vi "STAGE+mono+counter_edit24.vi"() -> ()   [LabVIEW 2017]
panel:
  out "Timeout":bool
  out "PROGRESS":sgl(slide) max=10 step=10 scale=0.0..1.0
  in  "?":enum32{"Scan Data", "Scans", "RT Data"}(tab)
  out "Spectrum":cluster{dbl[], dbl[]}(graph)
  out "Decay":cluster{dbl[], dbl[]}[](graph)
  in  "Collect Data!":bool
  out "Waveform Graph":waveform(dbl)[](graph)
  out "?":sgl(knob) scale=0.0..1000000.0
  out "Photon Counts":sgl
  in  "Wavelength":sgl
  in  "Show Real Time Data":bool
  in  "?":enum32{"DELAY", "COUNTER", "MONO", "PLOT"}(tab)
  in  "Data File Path":path
  out "Final time [ps]":sgl
  out "Current time [ps]":sgl
  out "Initial time [ps]":sgl
  in  "Set this as t0":bool
  in  "Axis":i64=1
  in  "Motor ON":bool
  in  "Motor OFF":bool
  out "Current Position [mm]":sgl
  out "Final Position [mm]":sgl
  in  "Data Points":sgl=100.0
  out "Current Point":sgl
  in  "Step Size [um]":sgl=10.0
  in  "Target [mm]":sgl format="%.3f"
  in  "Move":bool
  out "Initial position [mm]":sgl
  in  "GPIB address":string="23"
  in  "Count Mode":sgl(ring) items=["A,B for Preset T", "A-B for Preset T", "A+B for Preset T", "A for Preset B"]
  in  "Trigger mode":u16(ring) items=["10 MHz"=0, "Input 2"=2, "Input T"=3]
  in  "Channel A Input":sgl(ring)=1.0 items=["10 MHz", "Input 1"]
  in  "Channel B Input":u16(ring)=2 items=["Input 1"=1, "Input 2"=2]
  in  "Number of Measurements\n to take at one point/ Number of Periods":sgl=1.0 min=1 max=2000 step=1
  in  "Time between measurements\n at one point (s)/Dwell Time":sgl=0.002 min=0.002 max=60 step=0.001
  in  "gate mode (CW:0)":sgl(slide) scale=0.0..2.0 scale format="%.2f"
  out "Counts":sgl
  in  "Integrating time \nin 10^-7 sec":sgl=10000000.0
  in  "Discriminator Level (mV)":dbl min=-300.0 max=300.0 step=0.2
  in  "Discriminator Slope":bool
  in  "Channel":i16 min=0 max=2 step=1
  out "Current Units \n0=microns\n1=nanometers\n2=angstroms":dbl
  out "Grating #":sgl
  out "Blaze angle":sgl
  out "Grooves/mm":sgl
  out "Mono port":T1(ring)
  out "Time delay":sgl=450000.0 min=1
  in  "Step size":sgl=10.0 min=0
  in  "Scan to":sgl=4000.0
  in  "Scan from":sgl=2600.0
  out "Current wavelength":sgl
  in  "?":bool
  in  "NEW UNIT":T2(ring)
  in  "Array":sgl[](array[numeric])
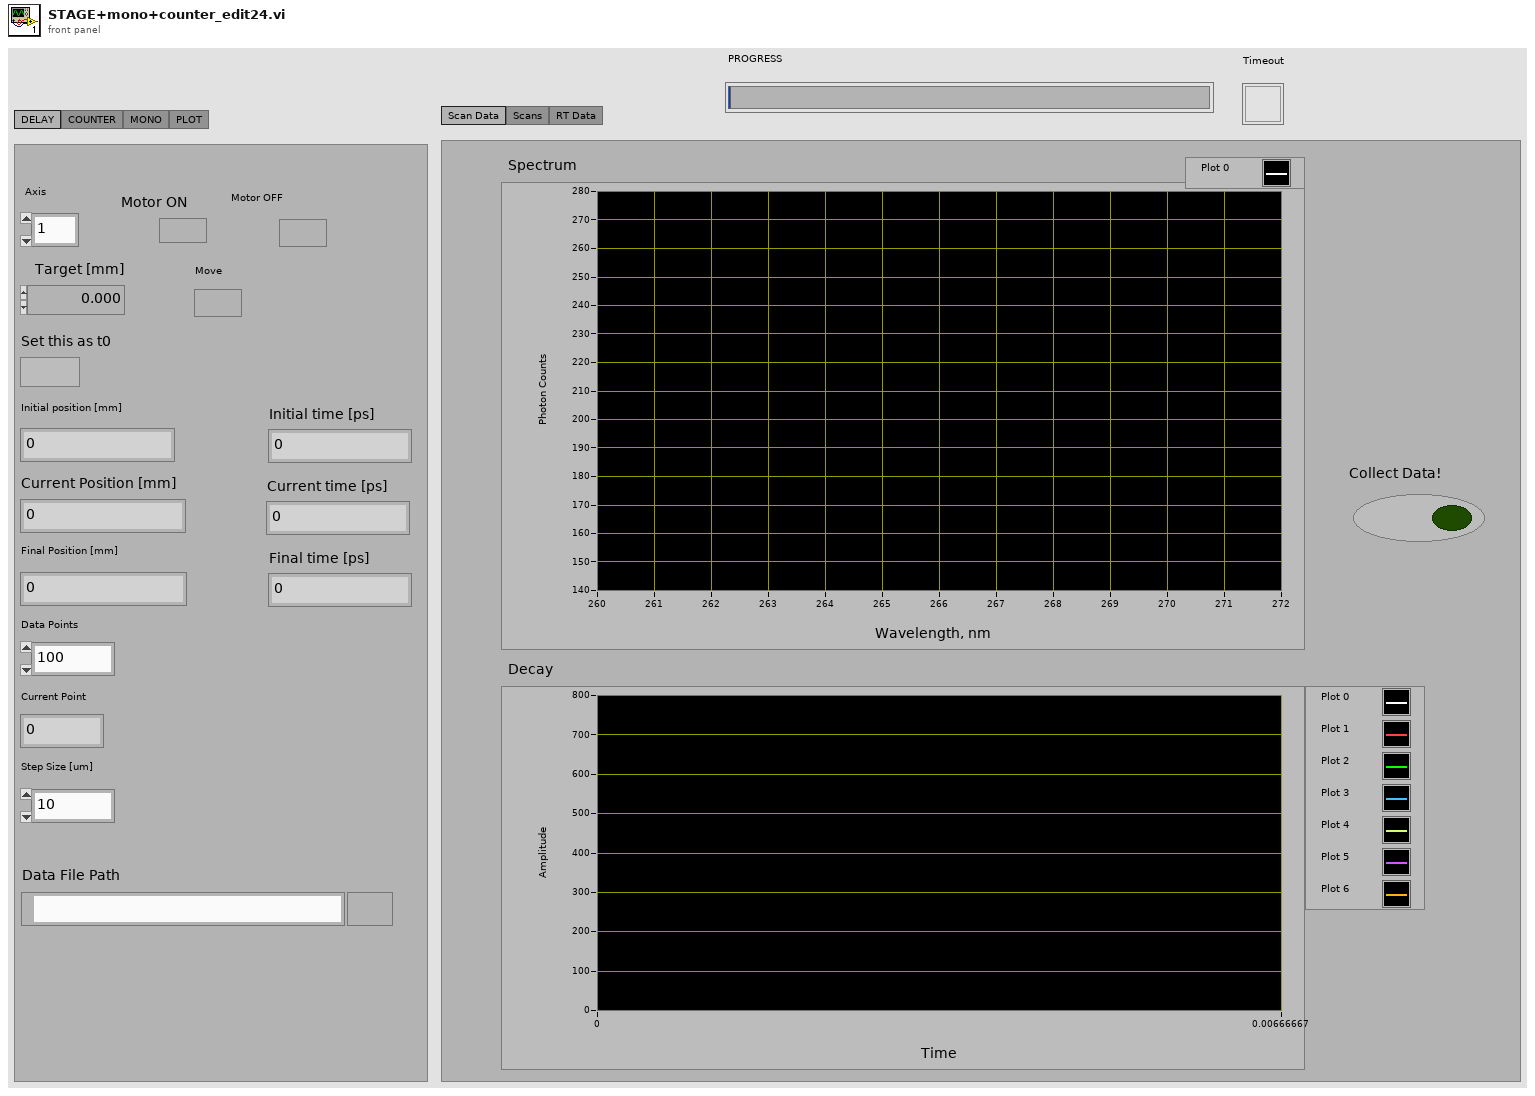
[diagram p1: front panel]
types:
  T1 = enum8{"COM 1", "COM 2", "COM 3", "COM 4", "COM 5", "COM 6", "COM 7", "COM 8", "COM 9"}
  T2 = enum16{"centi-Microns", " Nanometers", "   Angstroms"}
  T3 = cluster{"input XON/XOFF":bool, "input HW Handshake":bool, "input alt HW HShk":bool, "output XON/XOFF":bool, "output HW Handshake":bool, "output alt HW HShk":bool, "XOFF byte":u8, "XON byte":u8, "parity error byte":u16}
  T4 = enum16{"no parity", "odd parity", "even parity", "mark parity", "space parity"}
  T5 = enum16{"open", "replace", "create", "open or create", "replace or create", "replace or create with confirmation"}
  T6 = typedef "NI_Matrix.lvlib/RealMatrix.ctl" = dbl[][]
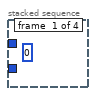
[diagram p2: hidden frame]
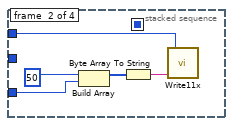
[diagram p3: hidden frame]
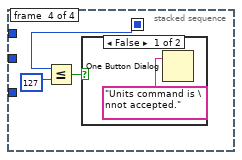
[diagram p4: hidden frame]
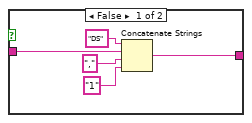
[diagram p7: hidden frame]
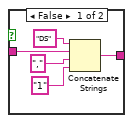
[diagram p9: hidden frame]
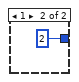
[diagram p13: hidden frame]
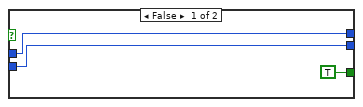
[diagram p14: hidden frame]
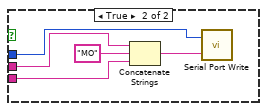
[diagram p15: hidden frame]
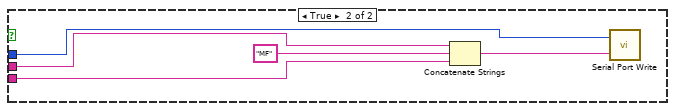
[diagram p16: hidden frame]
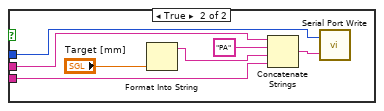
[diagram p17: hidden frame]
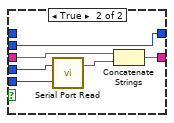
[diagram p19: hidden frame]
diagram:
  (unwired) FALSE
  w29 = u32 19200  # baud rate
  w28 = u16 8  # data bits
  w27 = enum16{"1 bit", "1.5 bits", "2 bits"}."1 bit"  # stop bits
  w31 = T4."no parity"  # parity
  w9 = 4  # 0=COM1 so n=COM(n+1)
  w30 = u16 1024  # buffer size
  n1 = flat-sequence {
    tunnel: [w34] -> w1
    tunnel: [w33] -> w2
    frame #0 {
      n2 = call "CM Com Read ini.vi"() -> ("Mono port"=w33:T1, "time delay1"=w34:u32)  [unwired: 7 in]
    }
  }
  n3 = call "CM Serial Port Setup.vi"("COM port"=w2, "time delay"=w1) -> ("time delay1"=w19:u32, "DK port Out"=w20:T1, "error code"=w22:i32)  [unwired: 7 in]
  n4 = Equal To 0?(x=w22) -> (x = 0?=w21:bool)
  n5 = case shown="True" w21 {
    tunnel: w20 -> [w37 w40]
    tunnel: w19 -> [w36 w39]
    tunnel: [w37 w40] -> w6
    tunnel: [w36 w39] -> w5
    tunnel: [TRUE FALSE] -> w4
    frame False {
    }
    frame True {
      n6 = call "CM Com Write ini.vi"("time delay1"=w40, "Mono port"=w39) -> ()  [unwired: 7 in]
      n7 = local write "Mono port"(w40) -> ()
      n8 = local write "Time delay"(w39) -> ()
    }
  }
  n9 = stacked-sequence {
    seq-local: [_ _ w48 _] -> [_ _ _ w55]
    tunnel: "NEW UNIT" -> [_ w42 _ _]
    tunnel: w2 -> [_ w41 w46 _]
    tunnel: w1 -> [_ _ w47 _]
    frame #0 {
      (unwired) u8 0
    }
    frame #1 {
      n10 = Build Array(u8 50, w42) -> (w44:u16[])
      n11 = Byte Array To String(unsigned byte array=w44) -> (string=w43:string)
      n12 = call "Write11x.vi"("string to write"=w43, "port number"=w41) -> ()  [unwired: 1 out]
    }
    frame #2 {
      n13 = call "Read11x.vi"("response size"=2, "timeout count"=w47, "port number"=w46) -> ("rcv index"=w49:u8[])  [unwired: 2 out]
      n14 = Index Array(array=w49, index=0) -> (element=w48:u8)
      n15 = Index Array(array=w49, index=1) -> ()  [unwired: 1 out]
    }
    frame #3 {
      n16 = Less Or Equal?(x=w55, y=127) -> (x <= y?=w53:bool)
      n17 = case shown="False" w53 {
        frame False {
          n18 = One Button Dialog(message="Units command is \nnot accepted.") -> ()  [unwired: 1 in, 1 out]
        }
        frame True {
        }
      }
    }
  }
  n19 = call <vilib>:"Serial Port Init.vi"("flow control etc."=T3 {"input XON/XOFF"=FALSE, "input HW Handshake"=FALSE, "input alt HW HShk"=FALSE, "output XON/XOFF"=FALSE, "output HW Handshake"=FALSE, "output alt HW HShk"=FALSE, "XOFF byte"=13, "XON byte"=11, "parity error byte"=0}, "parity"=w31, "buffer size"=w30, "stop bits"=w27, "data bits"=w28, "baud rate"=w29, "port number"=w9) -> ("error code"=w26:i32)
  n20 = Concatenate Strings("\r", "\n") -> (w23:string)
  n21 = while {
    tunnel: w5 -> [w59]
    tunnel: w6 -> [w58]
    stop <- TRUE continue-if-true
    n22 = case shown="True" "?" {
      tunnel: w59 -> [_ w62]
      tunnel: w58 -> [_ w61]
      frame False {
      }
      frame True {
        n23 = Two Button Dialog(message="Do you want to change grating?", 1:"No" ("F button name (\"Cancel\")"), 2:"Yes" ("T button name (\"OK\")")) -> (T button?=w63:bool)
        n24 = case shown="True" w63 {
          tunnel: w62 -> [_ w68]
          tunnel: w61 -> [_ w67]
          frame False {
          }
          frame True {
            n25 = Two Button Dialog(message="Disable voltage from PMT", 1:"Do not swich grating" ("F button name (\"Cancel\")"), 2:"Done" ("T button name (\"OK\")")) -> (T button?=w69:bool)
            n26 = case shown="True" w69 {
              tunnel: w68 -> [_ w81]
              tunnel: w67 -> [_ w80]
              frame False {
              }
              frame True {
                n27 = flat-sequence {
                  tunnel: w81 -> [w85]
                  tunnel: [w85] -> w75
                  tunnel: w80 -> [w84]
                  tunnel: [w84] -> w74
                  tunnel: [w82] -> w73
                  tunnel: w75 -> [w90]
                  tunnel: [w90] -> w78
                  tunnel: w74 -> [w91]
                  tunnel: [w91] -> w77
                  tunnel: w73 -> [w89]
                  tunnel: [w89] -> w76
                  tunnel: w78 -> [w95]
                  tunnel: w77 -> [w96]
                  tunnel: [w94] -> w79
                  tunnel: w76 -> [w94]
                  frame #0 {
                    n28 = local read "Grating #"() -> (w83:sgl)
                    n29 = case shown="2, Default" w83 {
                      tunnel: [1 2] -> w82
                      frame 2, Default {
                      }
                      frame 1 {
                      }
                    }
                    n30 = call "Select11x2.vi"("time delay"=w85, "NEW GRT?"=w82, "port number"=w84) -> ()  [unwired: 3 out]
                  }
                  frame #1 {
                    n31 = call "Query11x.vi"("port number"=w91, "QUERY"=u16 2, "time delay"=w90) -> ("STATUS MESSAGE"=w88:u16)  [unwired: 3 out]
                    n32 = local write "Grooves/mm"(w88) -> ()
                  }
                  frame #2 {
                    n33 = Divide(x=w95, y=i16 100 ("device (1)")) -> (x/y=w97:dbl)
                    n34 = call "Query11x.vi"("port number"=w96, "QUERY"=u16 3, "time delay"=w97) -> ("STATUS MESSAGE"=w93:u16)  [unwired: 3 out]
                    n35 = local write "Blaze angle"(w93) -> ()
                  }
                }
                n36 = local write "Grating #"(w79) -> ()
              }
            }
          }
        }
      }
    }
  }
  n37 = while {
    tunnel: w9 -> [w114]
    tunnel: w23 -> [w115]
    tunnel: w26 -> [_]
    tunnel: "Axis" -> [w112]
    stop <- TRUE continue-if-true
    w113 = u32 200  # timeout
    n38 = Format Into String(w112) -> (resulting string=w116:string)  [unwired: 3 in, 1 out]
    n39 = flat-sequence {
      tunnel: w116 -> [w121]
      tunnel: w115 -> [w120]
      tunnel: w114 -> [w122]
      tunnel: w113 -> [w119]
      tunnel: [w121] -> w111
      tunnel: [w120] -> w110
      tunnel: [w122] -> w109
      tunnel: [w119] -> w108
      tunnel: w111 -> [w132]
      tunnel: w110 -> [w131]
      tunnel: w109 -> [w133]
      tunnel: w108 -> [w129]
      tunnel: [w132] -> w107
      tunnel: [w131] -> w106
      tunnel: [w133] -> w105
      tunnel: [w129] -> w104
      tunnel: w107 -> [w142]
      tunnel: w106 -> [w141]
      tunnel: w105 -> [w143]
      tunnel: w104 -> [w139]
      tunnel: [w142] -> w103
      tunnel: [w141] -> w102
      tunnel: [w143] -> w101
      tunnel: [w139] -> w100
      tunnel: w103 -> [w155]
      tunnel: w102 -> [w152]
      tunnel: w101 -> [w154]
      tunnel: w100 -> [w153]
      frame #0 {
        n40 = case shown="False" "Motor ON" {
          tunnel: w122 -> [_ w128]
          tunnel: w121 -> [_ w125]
          tunnel: w120 -> [_ w124]
          frame False {
          }
          frame True {
            n41 = Concatenate Strings(w125, "MO" ("Substring"), w124) -> (w126:string)
            n42 = call <vilib>:"Serial Port Write.vi"("string to write"=w126, "port number"=w128) -> ()  [unwired: 1 out]
          }
        }
      }
      frame #1 {
        n43 = case shown="False" "Motor OFF" {
          tunnel: w133 -> [_ w138]
          tunnel: w132 -> [_ w135]
          tunnel: w131 -> [_ w134]
          frame False {
          }
          frame True {
            n44 = Concatenate Strings(w135, "MF" ("Substring"), w134) -> (w136:string)
            n45 = call <vilib>:"Serial Port Write.vi"("string to write"=w136, "port number"=w138) -> ()  [unwired: 1 out]
          }
        }
      }
      frame #2 {
        n46 = case shown="False" "Move" {
          tunnel: w143 -> [_ w150]
          tunnel: w142 -> [_ w147]
          tunnel: w141 -> [_ w146]
          frame False {
          }
          frame True {
            n47 = Format Into String("Target [mm]") -> (resulting string=w144:string)  [unwired: 3 in, 1 out]
            n48 = Concatenate Strings(w147, "PA" ("Substring"), w144, w146) -> (w148:string)
            n49 = call <vilib>:"Serial Port Write.vi"("string to write"=w148, "port number"=w150) -> ()  [unwired: 1 out]
          }
        }
      }
      frame #3 {
        n50 = case shown="True" "Set this as t0" {
          tunnel: w155 -> [_ w165]
          tunnel: w154 -> [_ w164]
          tunnel: w153 -> [_ w163]
          tunnel: w152 -> [_ w162]
          frame False {
          }
          frame True {
            n51 = flat-sequence {
              tunnel: w165 -> [w169]
              tunnel: w164 -> [w168]
              tunnel: [w168] -> w161
              tunnel: w163 -> [w166]
              tunnel: [w166] -> w160
              tunnel: w162 -> [w167]
              tunnel: w161 -> [w173]
              tunnel: [w173] -> w159
              tunnel: w160 -> [w172]
              tunnel: [w172] -> w158
              tunnel: [w174] -> w157
              tunnel: w159 -> [w179]
              tunnel: w158 -> [w177]
              tunnel: w157 -> [w176]
              tunnel: [w175] -> w156
              tunnel: w156 -> [w201]
              frame #0 {
                # "send position query"
                n52 = Concatenate Strings(w169, "TP" ("Substring"), w167) -> (w170:string)
                n53 = call <vilib>:"Serial Port Write.vi"("string to write"=w170, "port number"=w168) -> ()  [unwired: 1 out]
              }
              frame #1 {
                # "record current time"
                n54 = Tick Count (ms)() -> (millisecond timer value=w174:u32)
              }
              frame #2 {
                # "read characters in serial port"
                n55 = while {
                  shift-left: w176 -> [w180]
                  shift-right: [w181] -> _
                  tunnel: w177 -> [w184]
                  shift-left: "" -> [w187]
                  shift-right: [w186] -> w175
                  tunnel: w179 -> [w188]
                  stop <- w183 continue-if-true
                  n56 = Tick Count (ms)() -> (millisecond timer value=w182:u32)
                  n57 = call <vilib>:"Bytes At Serial Port.vi"("port number"=w188) -> ("byte count"=w189:u32)  [unwired: 1 out]
                  n58 = Subtract(x=w182, y=w180) -> (x-y=w185:u32)
                  n59 = Greater Than 0?(x=w189) -> (x > 0?=w190:bool)
                  n60 = Less?(x=w185, y=w184) -> (x < y?=w183:bool)
                  n61 = case shown="False" w190 {
                    tunnel: w189 -> [_ w198]
                    tunnel: w188 -> [_ w197]
                    tunnel: w187 -> [w192 w195]
                    tunnel: [w192 w194] -> w186
                    tunnel: [w191 w193] -> w181
                    tunnel: w182 -> [_ w193]
                    tunnel: w180 -> [w191 _]
                    frame False {
                    }
                    frame True {
                      n62 = call <vilib>:"Serial Port Read.vi"("requested byte count"=w198, "port number"=w197) -> ("string read"=w196:string)  [unwired: 1 out]
                      n63 = Concatenate Strings(w195, w196) -> (w194:string)
                    }
                  }
                }
              }
              frame #3 {
                n64 = Scan From String(input string=w201) -> (output 1=w199:dbl)  [unwired: 4 in, 3 out]
                n65 = Subtract(x=w199, y=w199) -> (x-y=→"Initial position [mm]":dbl)
              }
            }
          }
        }
      }
    }
    n66 = Wait Until Next ms Multiple(millisecond multiple=u32 50) -> ()  [unwired: 1 out]
  }
  n67 = while {
    tunnel: "GPIB address" -> [w205]
    tunnel: w6 -> [w204]
    tunnel: w5 -> [w203]
    tunnel: w4 -> [w202]
    stop <- TRUE continue-if-true
    n68 = case shown="True" "Show Real Time Data" {
      tunnel: w205 -> [_ w214]
      tunnel: w204 -> [_ w211]
      tunnel: w203 -> [_ w208]
      tunnel: w202 -> [_ w213]
      frame False {
      }
      frame True {
        n69 = flat-sequence {
          tunnel: w214 -> [w243]
          tunnel: "Wavelength" -> [w244]
          tunnel: [w244] -> w225
          tunnel: [w233] -> w224
          tunnel: [w234] -> w223
          tunnel: [w243] -> w222
          tunnel: w208 -> [w234]
          tunnel: w211 -> [w233]
          tunnel: w213 -> [_]
          tunnel: [w232] -> w209
          tunnel: w208 -> [w232]
          tunnel: [w252] -> w221
          tunnel: [w251] -> w220
          tunnel: [w249] -> w219
          tunnel: w225 -> [w247]
          tunnel: w224 -> [w252]
          tunnel: w223 -> [w251]
          tunnel: w222 -> [w249]
          tunnel: [w245] -> w210
          tunnel: w209 -> [w245]
          tunnel: w221 -> [_]
          tunnel: w220 -> [_]
          tunnel: w219 -> [w255]
          tunnel: [w255] -> w218
          tunnel: w211 -> [w254]
          tunnel: w210 -> [w253]
          tunnel: w218 -> [w264]
          tunnel: [w264] -> w217
          tunnel: w217 -> [w314]
          tunnel: [w314] -> w216
          tunnel: w216 -> [w315]
          tunnel: [w315] -> w215
          tunnel: w215 -> [w325]
          frame #0 {
            n70 = call "Query11x.vi"("port number"=w233, "QUERY"=sgl 4.0, "time delay"=w234) -> ("timeout"=w235:bool, "STATUS MESSAGE"=w236:u16)  [unwired: 2 out]
            n71 = call "Query11x.vi"("port number"=w233, "QUERY"=sgl 0.0, "time delay"=w234) -> ("timeout"=w230:bool, "STATUS MESSAGE"=w229:u16)  [unwired: 2 out]
            n72 = call "Query11x.vi"("port number"=w233, "QUERY"=sgl 2.0, "time delay"=w234) -> ("timeout"=w241:bool, "STATUS MESSAGE"=w240:u16)  [unwired: 2 out]
            n73 = call "Query11x.vi"("port number"=w233, "QUERY"=sgl 3.0, "time delay"=w234) -> ("timeout"=w239:bool, "STATUS MESSAGE"=w238:u16)  [unwired: 2 out]
            n74 = local write "Grating #"(w236) -> ()
            n75 = local write "Timeout"(w235) -> ()
            n76 = local write "Timeout"(w230) -> ()
            n77 = local write "Timeout"(w241) -> ()
            n78 = local write "Grooves/mm"(w240) -> ()
            n79 = local write "Timeout"(w239) -> ()
            n80 = local write "Blaze angle"(w238) -> ()
            n81 = Divide(x=w229, y=sgl 10.0 ("Numeric")) -> (x/y=w227:sgl)
            n82 = local write "Current wavelength"(w227) -> ()
          }
          frame #1 {
            n83 = Multiply(x=w247, y=1.0) -> (x*y=w246:dbl)
            n84 = call "Goto11x.vi"("time delay"=w251, "WAVELENGTH"=w246, "port number"=w252) -> ("timeout"=w250:bool)  [unwired: 2 out]
            n85 = local write "Timeout"(w250) -> ()
          }
          frame #2 {
            # "set counter time in 10^-7 seconds in CW"
            n86 = call "Query11x.vi"("port number"=w254, "QUERY"=sgl 0.0, "time delay"=w253) -> ("timeout"=w259:bool, "STATUS MESSAGE"=w258:u16)  [unwired: 2 out]
            n87 = local write "Timeout"(w259) -> ()
            n88 = Divide(x=w258, y=sgl 1.0) -> (x/y=w257:sgl)
            n89 = local write "Current wavelength"(w257) -> ()
          }
          frame #3 {
            # "Configures discriminator."
            n90 = flat-sequence {
              tunnel: w264 -> [w271]
              tunnel: [w271] -> w270
              tunnel: [w278] -> w269
              tunnel: [w276] -> w268
              tunnel: w263 -> [w277]
              tunnel: w270 -> [w276]
              tunnel: w265 -> [w275]
              tunnel: w269 -> [w297]
              tunnel: [w298] -> w267
              tunnel: w268 -> [w296]
              tunnel: [w296] -> w266
              tunnel: w265 -> [w294]
              tunnel: w267 -> [w310]
              tunnel: w266 -> [w309]
              tunnel: w261 -> [w304]
              tunnel: w265 -> [w303]
              frame #0 {
                # "Flush I/O buffers."
                n91 = for {
                  N: sgl 5.0 -> [_]
                  tunnel: w271 -> [w273]
                  n92 = GPIB Write(0:w273, 1:"\r") -> ()  [unwired: 3 in, 2 out]
                }
              }
              frame #1 {
                # "Set discriminator slope."
                n93 = case shown="True" w277 {
                  tunnel: [w284 w289] -> w279
                  tunnel: w275 -> [w283 w288]
                  frame False {
                    n94 = Concatenate Strings("DS", w283, ",", "1") -> (w284:string)
                  }
                  frame True {
                    n95 = Concatenate Strings("DS", w288, ",", "0") -> (w289:string)
                  }
                }
                n96 = GPIB Write(0:w276, 1:w279, 2:sgl 5.0) -> (6:w278:errorcluster)  [unwired: 2 in, 1 out]
              }
              frame #2 {
                # "Set discriminator mode to fixed."
                n97 = Concatenate Strings("DM", w294, ",", "0") -> (w293:string)
                n98 = GPIB Write(0:w296, 1:w293, 2:sgl 5.0, 3:w297) -> (6:w298:errorcluster)  [unwired: 1 in, 1 out]
              }
              frame #3 {
                # "Set discriminator level.\nMust be between +300 and -300 mV."
                n99 = Divide(x=w304, y=1000.0) -> (x/y=w312:dbl)
                n100 = Number To Fractional String(number=w312, precision (6)=sgl 4.0) -> (F-format string=w301:string)  [unwired: 2 in]
                n101 = Concatenate Strings("DL", w303, ",", w301) -> (w308:string)
                n102 = GPIB Write(0:w309, 1:w308, 2:sgl 5.0, 3:w310) -> (6:w305:errorcluster)  [unwired: 1 in, 1 out]
                n103 = call <vilib>:"General Error Handler.vi"("type of dialog (OK msg:1)"=sgl 1.0, "error in (no error)"=w305) -> ()  [unwired: 9 in, 5 out]
              }
            }
            n104 = local read "Channel"() -> (w262:i16)
            n105 = local read "Discriminator Slope"() -> (w263:bool)
            n106 = Number To Decimal String(number=w262) -> (decimal integer string=w265:string)  [unwired: 1 in]
            n107 = local read "Discriminator Level (mV)"() -> (w261:dbl)
          }
          frame #4 {
            n108 = call "Start.vi"("GPIB Address"=w314) -> ()  [unwired: 9 in]
          }
          frame #5 {
            # "Wait for Scan to Finish"
            n109 = for {
              N: sgl 1.0 -> [_]
              tunnel: w315 -> [w317]
              n110 = while {
                tunnel: w317 -> [w318]
                stop <- w320 stop-if-true
                n111 = call "ScanDone.vi"("Wait (ms)"=sgl 1000.0, "GPIB Address"=w318) -> ("Scan Finished?"=w320:bool)
              }
            }
          }
          frame #6 {
            n112 = call "Read Data.vi"("Channel Number"=sgl 0.0, "GPIB Address"=w325, "Number of Datapoints"=sgl 1.0) -> ("Data"=w326:i32[])
            n113 = property class="Knob (strict)"("Scale.Increment"=sgl 1000.0, "Scale.Maximum"=sgl 1000000.0, "Scale.Minimum"=sgl 0.0) -> ()  [unwired: 2 in, 2 out]
            n114 = Index Array(array=w326, index=sgl 0.0) -> (element=→"Photon Counts" →"?":i32)
          }
        }
      }
    }
  }
  n115 = while {
    tunnel: "Axis" -> [w338]
    tunnel: w9 -> [w337]
    tunnel: "GPIB address" -> [w336]
    tunnel: "Integrating time \nin 10^-7 sec" -> [w335]
    tunnel: w5 -> [w334]
    tunnel: w6 -> [w333]
    tunnel: w4 -> [w332]
    stop <- TRUE continue-if-true
    n116 = case shown="True" "Collect Data!" {
      selector: "Collect Data!" -> [_ w339]
      tunnel: w338 -> [_ w347]
      tunnel: w337 -> [_ w346]
      tunnel: w336 -> [_ w345]
      tunnel: w336 -> [_ w343]
      tunnel: w335 -> [_ w342]
      tunnel: w334 -> [_ w341]
      tunnel: w333 -> [_ w344]
      tunnel: w332 -> [_ w340]
      frame False {
      }
      frame True {
        n117 = flat-sequence {
          tunnel: w347 -> [w367]
          tunnel: w346 -> [w365]
          tunnel: w345 -> [w364]
          tunnel: w344 -> [w363]
          tunnel: w343 -> [w362]
          tunnel: w342 -> [w359]
          tunnel: w341 -> [w352]
          tunnel: w340 -> [w351]
          tunnel: w339 -> [_]
          frame #0 {
            w372 = 1000000000000.0
            w377 = sgl 1000.0
            w378 = sgl 300000000.0
            w384 = sgl 1.0
            n118 = Multiply(x="Step Size [um]", y="Data Points") -> (x*y=w381:sgl)
            n119 = Divide(x="Step Size [um]", y=1000.0) -> (x/y=w390:dbl)
            n120 = local read "Initial position [mm]"() -> (w369:sgl)
            n121 = Increment(x="Data Points") -> (x+1=w399:sgl)
            n122 = Multiply(x="Scan to", y=w384) -> (x*y=w358:sgl)
            n123 = Multiply(x="Scan from", y=w384) -> (x*y=w357:sgl)
            n124 = Divide(x=w381, y=sgl 1000.0) -> (x/y=w380:sgl)
            n125 = To Time Stamp(1:w357) -> (0:w387:timestamp)
            n126 = Multiply(x=w358, y=sgl 1.0) -> (x*y=w396:sgl)
            n127 = Multiply(x=sgl 1.0, y=w357) -> (x*y=w361:sgl)
            n128 = Divide(x=w390, y=1000.0) -> (x/y=w391:dbl)
            n129 = for {
              N: w399 -> [_]
              tunnel: w390 -> [w769]
              tunnel: w369 -> [w767]
              tunnel: [w760] -> w398 mode=indexing
              i -> [w768]
              # "distances"
              n130 = Multiply(x=w769, y=w768) -> (x*y=w766:dbl)
              n131 = Add(x=w767, y=w766) -> (x+y=w765:dbl)
              n132 = Divide(x=w765, y=sgl 1000.0) -> (x/y=w759:dbl)
              n133 = Divide(x=w759, y=sgl 300000000.0) -> (x/y=w762:dbl)
              n134 = Multiply(x=w762, y=1000000000000.0) -> (x*y=w760:dbl)
            }
            n135 = Subtract(x=w396, y=w361) -> (x-y=w402:sgl)
            n136 = Divide(x=w369, y=w377) -> (x/y=w375:sgl)
            n137 = Add(x=w369, y=w380) -> (x+y=w371:sgl)
            "Final Position [mm]" <- w371
            n138 = property on="Waveform Graph" class="WFGraph (strict)"("XScale.Increment"="Step size", "XScale.Maximum"=w358, "XScale.Minimum"=w357) -> ()  [unwired: 2 in, 2 out]
            n139 = Divide(x=w371, y=w377) -> (x/y=w376:sgl)
            n140 = Divide(x=w402, y="Step size") -> (x/y=w401:sgl)
            n141 = Divide(x=w375, y=w378) -> (x/y=w374:sgl)
            n142 = Divide(x=w391, y=sgl 300000000.0) -> (x/y=w393:dbl)
            n143 = Bundle By Name("Y"=dbl[] [], "t0"=w387, "dt"="Step size") -> (w386:waveform(dbl))  [unwired: 1 in]
            n144 = Divide(x=w376, y=w378) -> (x/y=w373:sgl)
            n145 = Multiply(x=w393, y=1000000000000.0) -> (x*y=w355:dbl)
            n146 = Multiply(x=w374, y=w372) -> (x*y=w354:dbl)
            "Initial time [ps]" <- w354
            n147 = Round Toward -Infinity(1:w401) -> (0:w360:sgl)
            n148 = Concatenate Strings("\r", "\n") -> (w366:string)
            n149 = Build Array(w386) -> (w350:waveform(dbl)[])
            n150 = Multiply(x=w373, y=w372) -> (x*y=w385:dbl)
            "Final time [ps]" <- w385
            n151 = Increment(x=w360) -> (x+1=w389:sgl)
            n152 = for {
              N: w389 -> [_]
              tunnel: "Step size" -> [w774]
              tunnel: w361 -> [w772]
              tunnel: [w770] -> _ mode=indexing
              i -> [w773]
              # "wavelengths"
              n153 = Multiply(x=w774, y=w773) -> (x*y=w771:sgl)
              n154 = Add(x=w772, y=w771) -> (x+y=w770:sgl)
            }
            n155 = for {
              N: "Data Points" -> [w426]
              tunnel: w369 -> [w467]
              tunnel: "Step Size [um]" -> [w463]
              tunnel: w367 -> [w460]
              tunnel: w366 -> [w457]
              tunnel: w365 -> [w458]
              tunnel: w364 -> [w456]
              tunnel: w363 -> [w454]
              tunnel: w362 -> [w455]
              tunnel: w361 -> [w417]
              tunnel: "Step size" -> [w449]
              tunnel: w360 -> [w448]
              tunnel: w359 -> [w447]
              tunnel: w358 -> [w412]
              tunnel: w357 -> [w411]
              tunnel: "Step size" -> [w413]
              tunnel: w355 -> [w428]
              tunnel: w354 -> [w445]
              shift-right: [w427] -> _
              shift-left: dbl[] [] -> [w423]
              tunnel: w352 -> [w440]
              tunnel: w363 -> [w439]
              tunnel: w351 -> [w438]
              shift-right: [w433] -> _
              shift-left: w350 -> [w434]
              shift-right: [w421] -> _
              shift-left: dbl[][] [] -> [w420]
              shift-right: [w409] -> _
              shift-left: dbl[][] [] -> [w407]
              i -> [w415]
              w437 = dbl[] []
              n156 = stacked-sequence {
                tunnel: w454 -> [w742]
                tunnel: w455 -> [_]
                frame #0 {
                  n157 = call <vilib>:"Close Serial Driver.vi"("port number"=w742) -> ()  [unwired: 1 out]
                  n158 = GPIB Misc(0:"loc 23" ("command string")) -> ()  [unwired: 1 in, 3 out]
                }
              }
              n159 = property on="Waveform Graph" class="WFGraph (strict)"("XScale.Increment"=w413, "XScale.Maximum"=w412, "XScale.Minimum"=w411) -> ()  [unwired: 2 in, 2 out]
              n160 = Number To Decimal String(number=w447) -> (decimal integer string=w452:string)  [unwired: 1 in]
              n161 = Divide(x=w463, y=sgl 1000.0) -> (x/y=w462:sgl)
              n162 = property on="PROGRESS" class="Slide (strict)"("Scale.Increment"=sgl 1.0, "Scale.Maximum"=w426, "Scale.Minimum"=sgl 0.0) -> ()  [unwired: 2 in, 2 out]
              n163 = Multiply(x=w428, y=w415) -> (x*y=w446:dbl)
              n164 = Add(x=sgl 1.0, y=w415) -> (x+y=→"PROGRESS":sgl)
              n165 = Concatenate Strings("CP 2,", w452) -> (w450:string)
              n166 = Add(x=w445, y=w446) -> (x+y=w424:dbl)
              n167 = Multiply(x=w462, y=w415) -> (x*y=w466:sgl)
              n168 = Add(x=w467, y=w466) -> (x+y=w465:sgl)
              n169 = Build Array (concatenate)(w423, w424) -> (w425:dbl[])
              n170 = Format Into String(w460) -> (resulting string=w459:string)  [unwired: 3 in, 1 out]
              n171 = GPIB Write(0:w456, 1:w450, 2:sgl 5.0 ("mode (0)")) -> ()  [unwired: 2 in, 2 out]
              n172 = flat-sequence {
                tunnel: w465 -> [w745]
                tunnel: [w745] -> w461
                tunnel: w457 -> [w747]
                tunnel: w459 -> [w746]
                tunnel: w458 -> [w743]
                tunnel: w461 -> [w756]
                tunnel: [w751] -> w410
                frame #0 {
                  n173 = Format Into String(w745) -> (resulting string=w744:string)  [unwired: 3 in, 1 out]
                  n174 = Wait (ms)(milliseconds to wait=sgl 100.0) -> ()  [unwired: 1 out]
                  n175 = Concatenate Strings(w746, "PA" ("Substring"), w744, w747) -> (w749:string)
                  n176 = call <vilib>:"Serial Port Write.vi"("string to write"=w749, "port number"=w743) -> ()  [unwired: 1 out]
                }
                frame #1 {
                  n177 = Divide(x=w756, y=sgl 1000.0) -> (x/y=w754:sgl)
                  n178 = Wait (ms)(milliseconds to wait=sgl 1000.0) -> ()  [unwired: 1 out]
                  n179 = Divide(x=w754, y=sgl 300000000.0) -> (x/y=w753:sgl)
                  n180 = Multiply(x=w753, y=1000000000000.0) -> (x*y=w751:dbl)
                  "Current time [ps]" <- w751
                  "Current Position [mm]" <- w756
                }
              }
              n181 = Add(x=w415, y=sgl 1.0) -> (x+y=w414:sgl)
              n182 = flat-sequence {
                tunnel: w456 -> [w493]
                tunnel: w417 -> [w492]
                tunnel: w449 -> [w491]
                tunnel: w448 -> [w490]
                tunnel: w412 -> [w489]
                tunnel: w411 -> [w488]
                tunnel: w437 -> [w487]
                tunnel: w437 -> [w486]
                tunnel: w413 -> [w485]
                tunnel: w440 -> [w484]
                tunnel: w439 -> [w483]
                tunnel: w438 -> [w482]
                tunnel: [w480] -> w436
                tunnel: [w481] -> _
                tunnel: [w480] -> w435
                tunnel: w414 -> [w479]
                tunnel: w410 -> [w478]
                tunnel: [w477] -> w408
                tunnel: w407 -> [w476]
                tunnel: w436 -> [w720]
                tunnel: [w723] -> w422
                tunnel: [w722] -> w419
                tunnel: [w721] -> w409
                tunnel: w408 -> [w721]
                frame #0 {
                  # "step size"
                  n183 = while {
                    tunnel: w493 -> [w535]
                    tunnel: w492 -> [w556]
                    tunnel: w491 -> [w528]
                    tunnel: w490 -> [w555]
                    tunnel: w489 -> [w531]
                    tunnel: w488 -> [w530]
                    tunnel: w485 -> [w532]
                    shift-right: [w552] -> w480
                    shift-left: w486 -> [w551]
                    shift-right: [w547] -> w481
                    shift-left: w487 -> [w554]
                    tunnel: w484 -> [w495]
                    tunnel: w483 -> [w494]
                    tunnel: w482 -> [w537]
                    tunnel: w479 -> [w516]
                    tunnel: w478 -> [w504]
                    shift-right: [w497] -> w477
                    shift-left: w476 -> [w496]
                    i -> [w524]
                    stop <- w526 stop-if-true
                    n184 = property on="Spectrum" class="XYGraph (strict)"("XScale.Increment"=w532, "XScale.Maximum"=w531, "XScale.Minimum"=w530) -> ()  [unwired: 2 in, 2 out]
                    n185 = Multiply(x=sgl 1.0, y=w528) -> (x*y=w527:sgl)
                    n186 = Multiply(x=w524, y=w527) -> (x*y=w557:sgl)
                    n187 = Greater Or Equal?(x=w524, y=w555) -> (x >= y?=w526:bool)
                    n188 = flat-sequence {
                      tunnel: w535 -> [w579]
                      tunnel: w536 -> [w580]
                      tunnel: [w580] -> w541
                      tunnel: [w560] -> w540
                      tunnel: [w561] -> w539
                      tunnel: [w579] -> w538
                      tunnel: w495 -> [w561]
                      tunnel: w494 -> [w560]
                      tunnel: w537 -> [_]
                      tunnel: [w578] -> w518
                      tunnel: w517 -> [w578]
                      tunnel: [w577] -> w505
                      tunnel: w504 -> [w577]
                      tunnel: w496 -> [w576]
                      tunnel: [w576] -> w503
                      tunnel: [w590] -> w546
                      tunnel: [w589] -> w545
                      tunnel: [w587] -> w544
                      tunnel: w541 -> [w583]
                      tunnel: w540 -> [w590]
                      tunnel: w539 -> [w589]
                      tunnel: w538 -> [w587]
                      tunnel: [w584] -> w519
                      tunnel: w518 -> [w584]
                      tunnel: [w583] -> w511
                      tunnel: [w582] -> w506
                      tunnel: w505 -> [w582]
                      tunnel: w503 -> [w581]
                      tunnel: [w581] -> w502
                      tunnel: w546 -> [_]
                      tunnel: w545 -> [_]
                      tunnel: w544 -> [w600]
                      tunnel: [w600] -> w534
                      tunnel: [w599] -> w520
                      tunnel: w519 -> [w599]
                      tunnel: [w598] -> w512
                      tunnel: w511 -> [w598]
                      tunnel: [w597] -> w507
                      tunnel: w506 -> [w597]
                      tunnel: w502 -> [w596]
                      tunnel: [w596] -> w501
                      tunnel: w494 -> [w595]
                      tunnel: w495 -> [w593]
                      tunnel: w494 -> [w594]
                      tunnel: w534 -> [w610]
                      tunnel: [w610] -> w533
                      tunnel: [w609] -> w521
                      tunnel: w520 -> [w609]
                      tunnel: [w608] -> w513
                      tunnel: w512 -> [w608]
                      tunnel: [w607] -> w508
                      tunnel: w507 -> [w607]
                      tunnel: w501 -> [w606]
                      tunnel: [w606] -> w500
                      tunnel: w533 -> [w667]
                      tunnel: [w667] -> w543
                      tunnel: [w666] -> w522
                      tunnel: w521 -> [w666]
                      tunnel: [w665] -> w514
                      tunnel: w513 -> [w665]
                      tunnel: [w664] -> w509
                      tunnel: w508 -> [w664]
                      tunnel: w500 -> [w663]
                      tunnel: [w663] -> w499
                      tunnel: w543 -> [w672]
                      tunnel: [w672] -> w542
                      tunnel: [w671] -> w523
                      tunnel: w522 -> [w671]
                      tunnel: [w670] -> w515
                      tunnel: w514 -> [w670]
                      tunnel: [w669] -> w510
                      tunnel: w509 -> [w669]
                      tunnel: w499 -> [w668]
                      tunnel: [w668] -> w498
                      tunnel: [w683] -> w549
                      tunnel: w542 -> [w715]
                      tunnel: w523 -> [w681]
                      tunnel: w516 -> [w684]
                      tunnel: w515 -> [w685]
                      tunnel: w510 -> [w687]
                      tunnel: w498 -> [w682]
                      tunnel: [w680] -> w497
                      frame #0 {
                        n189 = call "Query11x.vi"("port number"=w560, "QUERY"=sgl 2.0, "time delay"=w561) -> ("timeout"=w569:bool, "STATUS MESSAGE"=→"Grooves/mm":u16)  [unwired: 2 out]
                        n190 = call "Query11x.vi"("port number"=w560, "QUERY"=sgl 0.0, "time delay"=w561) -> ("timeout"=w574:bool, "STATUS MESSAGE"=w573:u16)  [unwired: 2 out]
                        n191 = call "Query11x.vi"("port number"=w560, "QUERY"=sgl 4.0, "time delay"=w561) -> ("timeout"=w564:bool, "STATUS MESSAGE"=→"Grating #":u16)  [unwired: 2 out]
                        n192 = call "Query11x.vi"("port number"=w560, "QUERY"=14.0, "time delay"=w561) -> ("STATUS MESSAGE"=→"Current Units \n0=microns\n1=nanometers\n2=angstroms":u16)  [unwired: 3 out]
                        n193 = call "Query11x.vi"("port number"=w560, "QUERY"=sgl 3.0, "time delay"=w561) -> ("timeout"=w567:bool, "STATUS MESSAGE"=→"Blaze angle":u16)  [unwired: 2 out]
                        n194 = local write "Timeout"(w574) -> ()
                        n195 = Divide(x=w573, y=1 ("Numeric")) -> (x/y=→"Current wavelength":dbl)
                        n196 = local write "Timeout"(w569) -> ()
                        n197 = local write "Timeout"(w564) -> ()
                        n198 = local write "Timeout"(w567) -> ()
                      }
                      frame #1 {
                        n199 = Multiply(x=w583, y=sgl 1.0) -> (x*y=w585:sgl)
                        n200 = call "Goto11x.vi"("time delay"=w589, "WAVELENGTH"=w585, "port number"=w590) -> ("timeout"=w588:bool)  [unwired: 2 out]
                        n201 = local write "Timeout"(w588) -> ()
                      }
                      frame #2 {
                        # "set counter time in 10^-7 seconds in CW"
                        n202 = call "Query11x.vi"("port number"=w595, "QUERY"=sgl 0.0, "time delay"=w593) -> ("timeout"=w604:bool, "STATUS MESSAGE"=w603:u16)  [unwired: 2 out]
                        n203 = call "Query11x.vi"("port number"=w594, "QUERY"=14.0, "time delay"=w593) -> ("STATUS MESSAGE"=w591:u16)  [unwired: 3 out]
                        n204 = local write "Timeout"(w604) -> ()
                        n205 = Divide(x=w603, y=sgl 1.0) -> (x/y=w602:sgl)
                        n206 = local write "Current wavelength"(w602) -> ()
                        n207 = local write "Current Units \n0=microns\n1=nanometers\n2=angstroms"(w591) -> ()
                      }
                      frame #3 {
                        # "Configures discriminator."
                        n208 = flat-sequence {
                          tunnel: w610 -> [w620]
                          tunnel: [w620] -> w619
                          tunnel: [w627] -> w618
                          tunnel: [w625] -> w617
                          tunnel: "Discriminator Slope" -> [w626]
                          tunnel: w619 -> [w625]
                          tunnel: w611 -> [w624]
                          tunnel: w618 -> [w646]
                          tunnel: [w647] -> w616
                          tunnel: w617 -> [w645]
                          tunnel: [w645] -> w615
                          tunnel: w611 -> [w643]
                          tunnel: w616 -> [w659]
                          tunnel: w615 -> [w658]
                          tunnel: "Discriminator Level (mV)" -> [w653]
                          tunnel: w611 -> [w652]
                          frame #0 {
                            # "Flush I/O buffers."
                            n209 = for {
                              N: sgl 5.0 -> [_]
                              tunnel: w620 -> [w622]
                              n210 = GPIB Write(0:w622, 1:"\r") -> ()  [unwired: 3 in, 2 out]
                            }
                          }
                          frame #1 {
                            # "Set discriminator slope."
                            n211 = case shown="True" w626 {
                              tunnel: [w633 w638] -> w628
                              tunnel: w624 -> [w632 w637]
                              frame False {
                                n212 = Concatenate Strings("DS", w632, ",", "1") -> (w633:string)
                              }
                              frame True {
                                n213 = Concatenate Strings("DS", w637, ",", "0") -> (w638:string)
                              }
                            }
                            n214 = GPIB Write(0:w625, 1:w628, 2:sgl 5.0) -> (6:w627:errorcluster)  [unwired: 2 in, 1 out]
                          }
                          frame #2 {
                            # "Set discriminator mode to fixed."
                            n215 = Concatenate Strings("DM", w643, ",", "0") -> (w642:string)
                            n216 = GPIB Write(0:w645, 1:w642, 2:sgl 5.0, 3:w646) -> (6:w647:errorcluster)  [unwired: 1 in, 1 out]
                          }
                          frame #3 {
                            # "Set discriminator level.\nMust be between +300 and -300 mV."
                            n217 = Divide(x=w653, y=1000.0) -> (x/y=w661:dbl)
                            n218 = Number To Fractional String(number=w661, precision (6)=sgl 4.0) -> (F-format string=w650:string)  [unwired: 2 in]
                            n219 = Concatenate Strings("DL", w652, ",", w650) -> (w657:string)
                            n220 = GPIB Write(0:w658, 1:w657, 2:sgl 5.0, 3:w659) -> (6:w654:errorcluster)  [unwired: 1 in, 1 out]
                            n221 = call <vilib>:"General Error Handler.vi"("type of dialog (OK msg:1)"=1, "error in (no error)"=w654) -> ()  [unwired: 9 in, 5 out]
                          }
                        }
                        n222 = Number To Decimal String(number="Channel") -> (decimal integer string=w611:string)  [unwired: 1 in]
                      }
                      frame #4 {
                        n223 = call "Start.vi"("GPIB Address"=w667) -> ()  [unwired: 9 in]
                      }
                      frame #5 {
                        # "Wait for Scan to Finish"
                        n224 = for {
                          N: sgl 1.0 -> [_]
                          tunnel: w672 -> [w674]
                          n225 = while {
                            tunnel: w674 -> [w675]
                            stop <- w677 stop-if-true
                            n226 = call "ScanDone.vi"("Wait (ms)"=1000, "GPIB Address"=w675) -> ("Scan Finished?"=w677:bool)
                          }
                        }
                      }
                      frame #6 {
                        w686 = sgl 0.0
                        w694 = "\r\n"
                        n227 = call "Read Data.vi"("Channel Number"=sgl 0.0, "GPIB Address"=w715, "Number of Datapoints"=sgl 1.0) -> ("Data"=w716:i32[])
                        n228 = Index Array(array=w716, index=sgl 0.0) -> (element=w683:i32)
                        "Counts" <- w683
                        n229 = local read "Integrating time \nin 10^-7 sec"() -> (w692:sgl)
                        n230 = Replace Array Subset(array=w682, new element #1=w683, index (row) #1=w681, index (col) #1=w684, new element #2=w685, index (row) #2=w681, index (col) #2=w686, new element #3=w687, index (row) #3=w686, index (col) #3=w684) -> (w680:T6)
                        n231 = Array To Spreadsheet String(delimiter (Tab)=",", array=w680, 3:"%f" ("format string")) -> (spreadsheet string=w693:string)
                        n232 = local read "Blaze angle"() -> (w710:sgl)
                        n233 = local read "Grating #"() -> (w709:sgl)
                        n234 = Multiply(x=w692, y=1e-07) -> (x*y=w691:dbl)
                        n235 = Get Date/Time In Seconds() -> (seconds since 1Jan1904=w704:timestamp)
                        n236 = Format Date/Time String(time format string (%c)="%Y-%b-%d %H:%M:%S", seconds (now)=w704) -> (date/time string=w705:string)  [unwired: 1 in]
                        n237 = Number To Decimal String(number=w691) -> (decimal integer string=w706:string)  [unwired: 1 in]
                        n238 = Number To Decimal String(number=w709) -> (decimal integer string=w707:string)  [unwired: 1 in]
                        n239 = Number To Decimal String(number=w710) -> (decimal integer string=w695:string)  [unwired: 1 in]
                        n240 = call <vilib>:"Space Constant.vi"() -> ("String"=w708:string)
                        n241 = Open/Create/Replace File(file path (use dialog)="Data File Path", operation (0:open)=T5."replace or create") -> (refnum out=w714:refnum<file>)  [unwired: 4 in, 2 out]
                        n242 = Concatenate Strings(w694, "Data was taken on ", w705, w694, "Integration Time is ", w706, w708, "s", w694, "Monochromator gratng # ", w707, "; ", "blazed for ", w695, w708, "nm", w694, w694, w694, w693) -> (w689:string)
                        n243 = Write to Text File(file (use dialog)=w714, text=w689) -> (refnum out=w679:refnum<file>)  [unwired: 2 in, 2 out]
                        n244 = Flush File(refnum=w679) -> (refnum out=w678:refnum<file>)  [unwired: 1 in, 1 out]
                        n245 = Close File(refnum=w678) -> ()  [unwired: 1 in, 2 out]
                      }
                    }
                    n246 = Add(x=w557, y=w556) -> (x+y=w536:sgl)
                    n247 = Add(x=w524, y=sgl 1.0) -> (x+y=w517:sgl)
                    n248 = Build Array (concatenate)(w554, w536) -> (w553:dbl[])
                    n249 = Build Array (concatenate)(w551, w549) -> (w550:dbl[])
                    n250 = Bundle(w553, w550) -> (w548:cluster{dbl[], dbl[]})  [unwired: 1 in]
                    "Spectrum" <- w548
                    n251 = Unbundle(w548) -> (w547:dbl[], w552:dbl[])
                  }
                }
                frame #1 {
                  n252 = Array Size(array="Array") -> (size(s)=w722:i32)
                  n253 = flat-sequence {
                    tunnel: w720 -> [w729]
                    tunnel: "Array" -> [w728]
                    tunnel: w722 -> [w727]
                    tunnel: [w725] -> w723
                    frame #0 {
                      n254 = for {
                        N: w727 -> [_]
                        tunnel: w728 -> [w740]
                        tunnel: w729 -> [w735]
                        shift-right: [w730] -> w725
                        shift-left: dbl[] [] -> [w731]
                        i -> [w733]
                        n255 = local read "Scan from"() -> (w738:sgl)
                        n256 = Index Array(array=w740, index=w733) -> (element=w739:sgl)
                        n257 = local read "Step size"() -> (w736:sgl)
                        n258 = Subtract(x=w739, y=w738) -> (x-y=w737:sgl)
                        n259 = Divide(x=w737, y=w736) -> (x/y=w734:sgl)
                        n260 = Index Array(array=w735, index=w734) -> (element=w732:dbl)
                        n261 = Insert Into Array(array=w731, index=w733, new element=w732) -> (w730:dbl[])
                      }
                    }
                  }
                }
              }
              n262 = local read "Scan from"() -> (w431:sgl)
              n263 = local read "Step size"() -> (w429:sgl)
              n264 = To Time Stamp(1:w431) -> (0:w430:timestamp)
              n265 = Bundle By Name("Y"=w435, "t0"=w430, "dt"=w429) -> (w432:waveform(dbl))  [unwired: 1 in]
              n266 = Build Array (concatenate)(w434, w432) -> (w433:waveform(dbl)[])
              "Waveform Graph" <- w433
              n267 = for {
                N: w419 -> [_]
                tunnel: [w475] -> w427
                tunnel: w425 -> [w474]
                tunnel: w422 -> [w472]
                tunnel: [w471] -> w421
                tunnel: w420 -> [w473]
                tunnel: [w468] -> w418 mode=indexing
                i -> [w470]
                n268 = Build Array (concatenate)(w473, w472) -> (w471:dbl[][])
                n269 = Index Array(array=w472, index=w470) -> ()  [unwired: 1 out]
                n270 = Index Array(array=w471, index (col)=w470) -> (element=w469:dbl[])  [unwired: 1 in]
                n271 = Bundle(w474, w469) -> (w468:cluster{dbl[], dbl[]})  [unwired: 1 in]
                n272 = Unbundle(w468) -> (w475:dbl[])  [unwired: 1 out]
              }
              "Decay" <- w418
              "Current Point" <- w415
            }
            n273 = property on="Decay" class="XYGraph (strict)"("XScale.Increment"=w355, "XScale.Maximum"=w385, "XScale.Minimum"=w354) -> ()  [unwired: 2 in, 2 out]
            n274 = Build Array (concatenate)(sgl 0.0, w398) -> ()  [unwired: 1 out]
          }
        }
      }
    }
  }
  n275 = call "Configure.vi"("Dwell Time (s)"="Time between measurements\n at one point (s)/Dwell Time", "Channel T Input"="Trigger mode", "Channel B Input"="Channel B Input", "Channel A Input"="Channel A Input", "Integrating time, 10^-7 sec"="Integrating time \nin 10^-7 sec", "gate mode (CW:0)"="gate mode (CW:0)", "Scan End Mode"=FALSE, "Number of Periods"="Number of Measurements\n to take at one point/ Number of Periods", "Count Mode"="Count Mode", "GPIB Address"="GPIB address") -> ()
  "Mono port" <- w2
  "Time delay" <- w1
